vi "write.vi"(8 "error in (no error)":errorcluster, 10 "data":string, 11 "Device in":T1) -> (0 "error out":errorcluster, 3 "Device out":T1)   [LabVIEW 2016]
uses:
  device.ctl
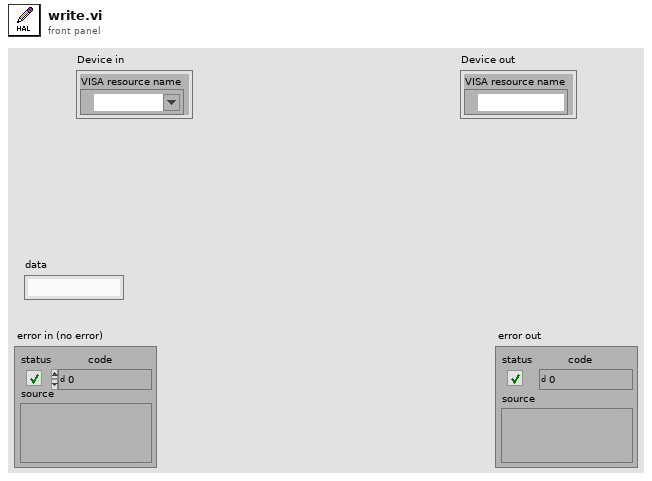
[diagram p1: front panel]
types:
  T1 = typedef "device.ctl" = cluster{"VISA resource name":refnum<visa-resource-name>}
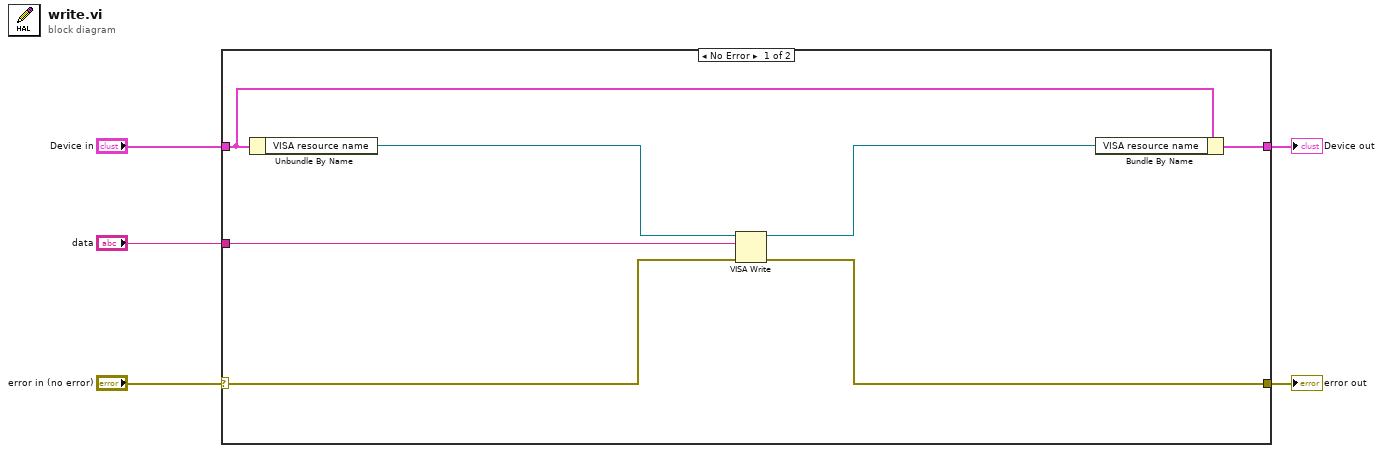
[diagram p0: block diagram]
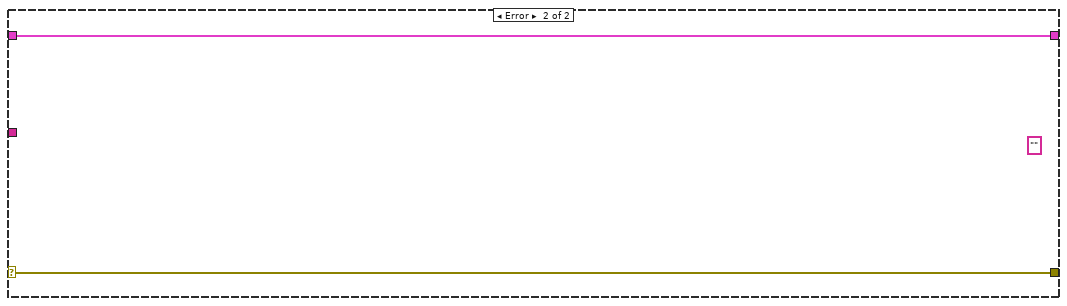
[diagram p2: hidden frame]
diagram:
  n1 = case shown="No Error" "error in (no error)" {
    selector: "error in (no error)" -> [w12 w13]
    tunnel: [w7 w14] -> w4
    tunnel: "Device in" -> [w8 w14]
    tunnel: [w11 w13] -> w2
    tunnel: "data" -> [w9 _]
    frame No Error {
      n2 = Unbundle By Name(w8) -> ("VISA resource name"=w6:refnum<visa-resource-name>)
      n3 = VISA Write(VISA resource name=w6, write buffer=w9, error in (no error)=w12) -> (VISA resource name out=w10:refnum<visa-resource-name>, error out=w11:errorcluster)  [unwired: 1 out]
      n4 = Bundle By Name(cluster=w8, "VISA resource name"=w10) -> (w7:T1)
    }
    frame Error {
      (unwired) "" ("read buffer")
    }
  }
  "error out" <- w2
  "Device out" <- w4
